vi "test_brokenVITest.vi"(8 "error in (no error)":errorcluster, 11 "TestCase in":refnum<class "lvCICD_TestCase.lvclass">) -> (0 "error out":errorcluster, 3 "TestCase out":refnum<class "lvCICD_TestCase.lvclass">)   [LabVIEW 2019, in "lvCICD_TestCase.lvclass"]
uses:
  lvCICD_TestCase.lvclass
  <vilib>/addons/_JKI Toolkits/VI Tester/TestCase.llb/TestCase.lvclass
  C:/Program Files (x86)/National Instruments/LabVIEW 2019/vi.lib/addons/_JKI Toolkits/VI Tester/TestCase.llb/TestCase.lvclass
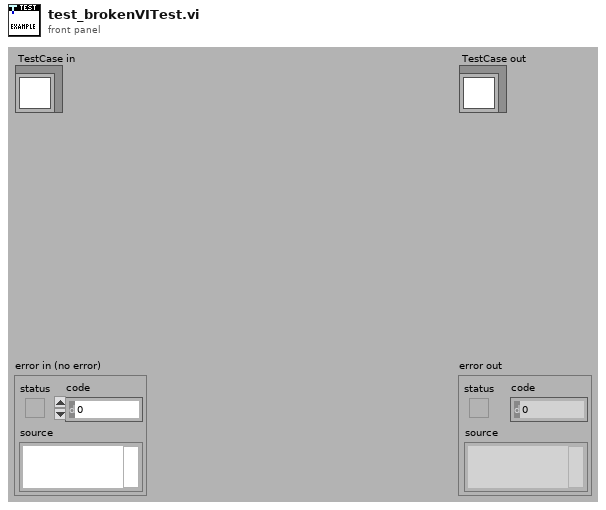
[diagram p1: front panel]
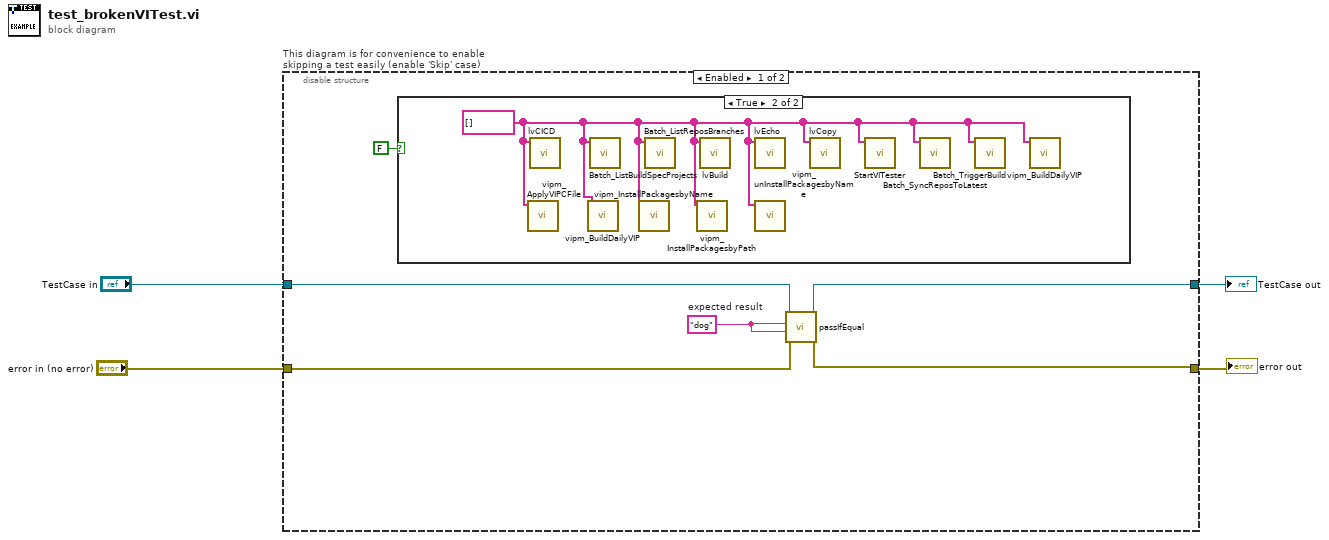
[diagram p0: block diagram]
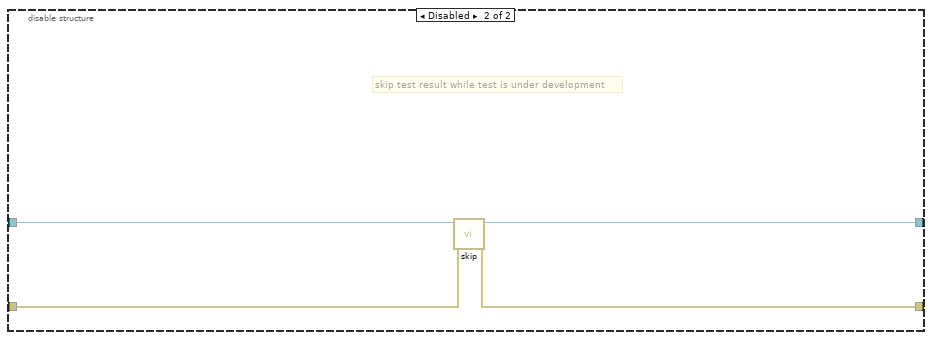
[diagram p3: hidden frame]
diagram:
  n1 = disable-structure "This diagram is for convenience to enable skipping a test easily (enable 'Skip' case)" shown="Enabled" {
    disable-tunnel: "TestCase in" -> [w10 w15]
    disable-tunnel: [w9 w13] -> w1
    disable-tunnel: [w8 w14] -> w3
    disable-tunnel: "error in (no error)" -> [w7 w12]
    frame Enabled {
      w6 = "dog"  # expected result
      n2 = case shown="True" FALSE {
        frame False {
        }
        frame True {
          w11 = string[] [] ("CommandLine")
          n3 = call "vipm_ApplyVIPCFile.vi"("CommandLine"=w11) -> ()  [unwired: 9 in, 2 out]
          n4 = call "lvCICD.vi"("CommandLine"=w11) -> ()  [unwired: 9 in, 2 out]
          n5 = call "vipm_BuildDailyVIP.vi"("CommandLine"=w11) -> ()  [unwired: 9 in, 2 out]
          n6 = call "Batch_ListBuildSpecProjects.vi"("CommandLine"=w11) -> ()  [unwired: 9 in, 2 out]
          n7 = call "vipm_InstallPackagesbyName.vi"("CommandLine"=w11) -> ()  [unwired: 9 in, 2 out]
          n8 = call "Batch_ListReposBranches.vi"("CommandLine"=w11) -> ()  [unwired: 9 in, 2 out]
          n9 = call "vipm_InstallPackagesbyPath.vi"("CommandLine"=w11) -> ()  [unwired: 9 in, 2 out]
          n10 = call "lvBuild.vi"("CommandLine"=w11) -> ()  [unwired: 9 in, 2 out]
          n11 = call "lvEcho.vi"("CommandLine"=w11) -> ()  [unwired: 9 in, 2 out]
          n12 = call "vipm_unInstallPackagesbyName.vi"("CommandLine"=w11) -> ()  [unwired: 9 in, 2 out]
          n13 = call "lvCopy.vi"("CommandLine"=w11) -> ()  [unwired: 9 in, 2 out]
          n14 = call "StartVITester.vi"("CommandLine"=w11) -> ()  [unwired: 9 in, 2 out]
          n15 = call "Batch_SyncReposToLatest.vi"("CommandLine"=w11) -> ()  [unwired: 9 in, 2 out]
          n16 = call "Batch_TriggerBuild.vi"("CommandLine"=w11) -> ()  [unwired: 9 in, 2 out]
          n17 = call "vipm_BuildDailyVIP.vi"("CommandLine"=w11) -> ()  [unwired: 9 in, 2 out]
        }
      }
      n18 = call-dynamic "passIfEqual.vi"("error in (no error)"=w7, "y"=w6, "x"=w6, "TestCase in"=w10) -> ("error out"=w8:errorcluster, "TestCase out"=w9:refnum<class "lvCICD_TestCase.lvclass">)  [unwired: 6 in]
    }
    frame Disabled {
      # "skip test result while test is under development"
      n19 = call <vilib>:"skip.vi"("error in (no error)"=w12, "TestCase in"=w15) -> ("error out"=w14:errorcluster, "TestCase out"=w13:refnum<class "lvCICD_TestCase.lvclass">)  [unwired: 8 in]
    }
  }
  "error out" <- w3
  "TestCase out" <- w1
